vi "WPI_SerialPortGetPortName.vi"(8 "error in (no error)":errorcluster, 11 "Serial Port":T1) -> (0 "error out":errorcluster, 3 "VISA Refnum out":refnum<visa-resource-name>)   [LabVIEW 2017]
uses:
  <vilib>/Rock Robotics/WPI/SerialPort/WPI_SerialPort.ctl
panel:
  out "Hub Path":string[](array[string])
  out "OS Resource":string[](array[string])
  out "VISA Resource":string[](array[string])
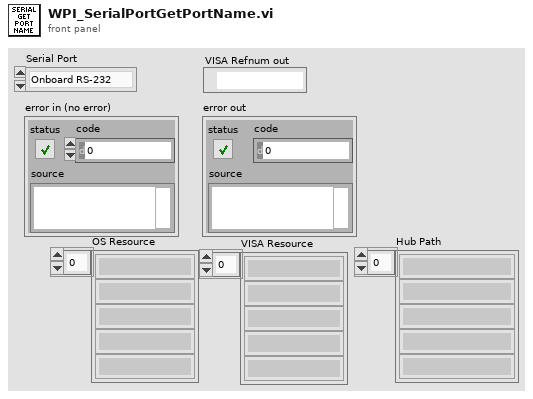
[diagram p1: front panel]
types:
  T1 = typedef "WPI_SerialPort.ctl" = enum16{"Onboard RS-232", "MXP TTL", "USB 1", "USB 2"}
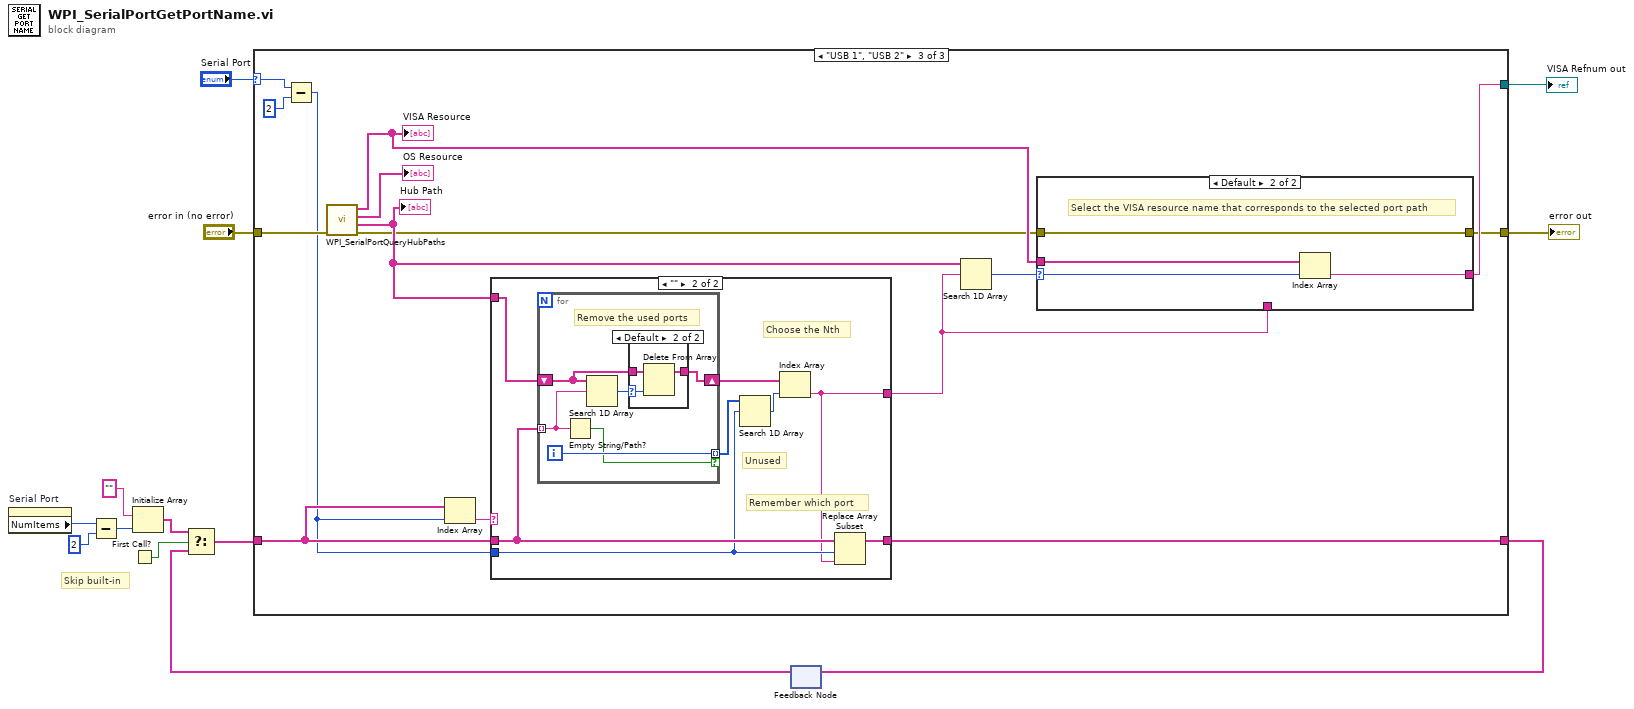
[diagram p0: block diagram]
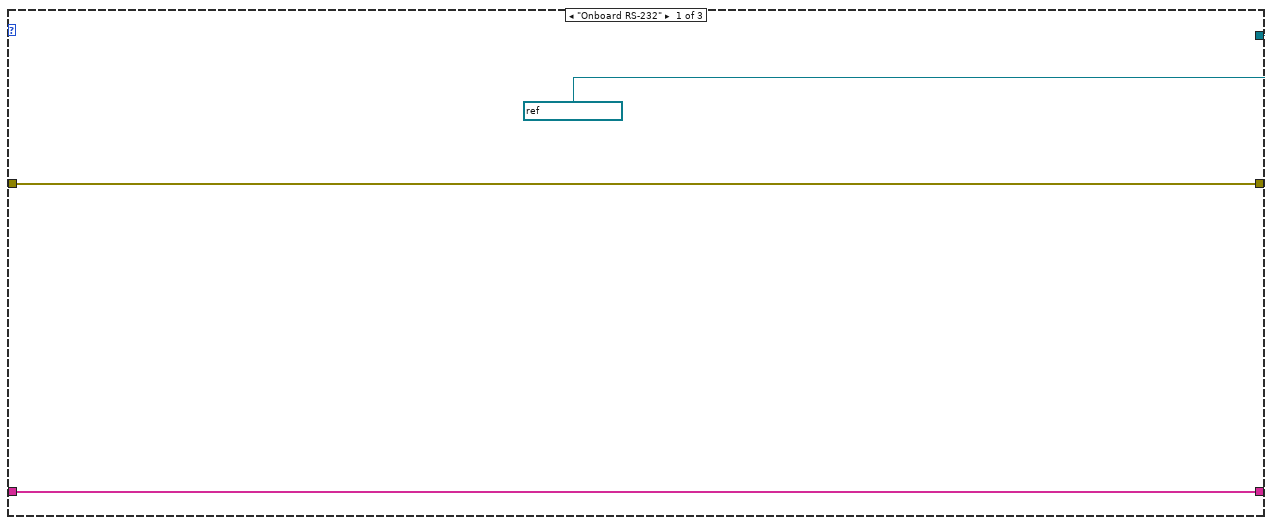
[diagram p2: hidden frame]
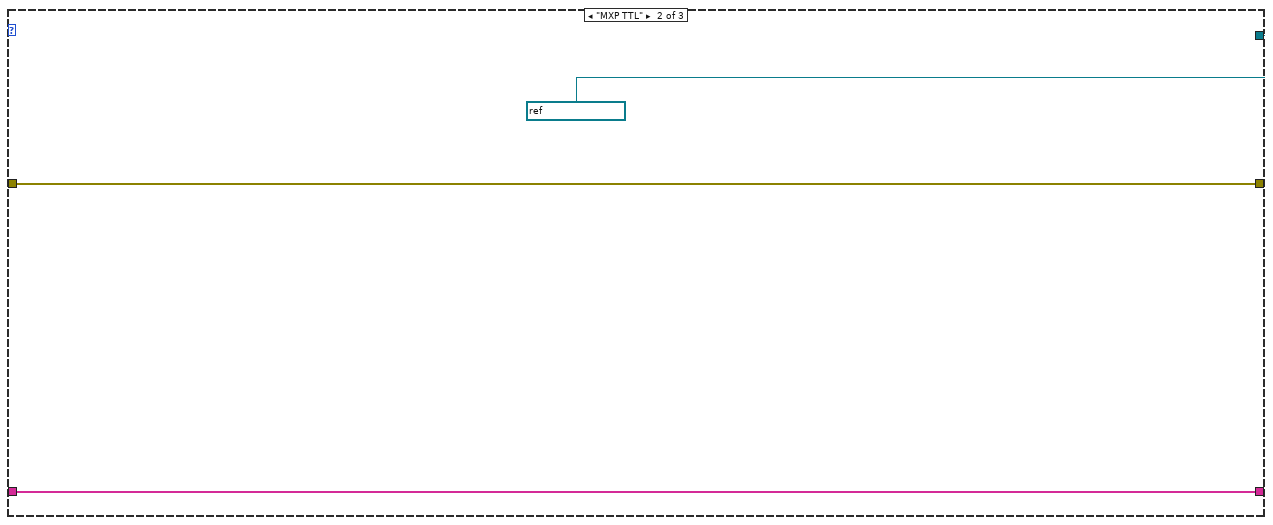
[diagram p3: hidden frame]
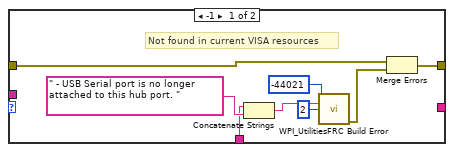
[diagram p4: hidden frame]
diagram:
  # "Skip built-in"
  n1 = property on="Serial Port" class="Enum (strict)"() -> ("NumItems"=w9:u32)  [unwired: 2 in, 2 out]
  n2 = Subtract(x=w9, y=u32 2 ("x")) -> (x-y=w2:u32)
  n3 = First Call?() -> (First Call?: T/F=w6:bool)
  n4 = Initialize Array("", w2) -> (w7:string[])
  n5 = feedback #1() -> (w5:string[])  [unwired: 1 in]
  n6 = Select(t=w7, s=w6, f=w5) -> (s? t:f=w4:string[])
  n7 = case shown="\"USB 1\", \"USB 2\"" "Serial Port" {
    selector: "Serial Port" -> [_ _ w29]
    tunnel: [refnum<visa-resource-name> "ASRL1::INSTR" ("VISA resource name") refnum<visa-resource-name> "ASRL2::INSTR" ("VISA resource name") w23] -> w13
    tunnel: "error in (no error)" -> [w15 w18 w34]
    tunnel: [w15 w18 w21] -> w10
    tunnel: w4 -> [w14 w17 w31]
    tunnel: [w14 w17 w27] -> w3
    frame "Onboard RS-232" {
    }
    frame "MXP TTL" {
    }
    frame "USB 1", "USB 2" {
      n8 = Subtract(x=w29, y=2 ("x")) -> (x-y=w28:i32)
      n9 = call <vilib>:"WPI_SerialPortQueryHubPaths.vi"("error in (no error)"=w34) -> ("error out"=w22:errorcluster, "Hub Path"=w26:string[], "OS Resource"=→"OS Resource":string[], "VISA Resource"=w24:string[])  [unwired: 7 in]
      "VISA Resource" <- w24
      "Hub Path" <- w26
      n10 = Index Array(array=w31, index=w28) -> (element=w32:string)
      n11 = case shown="\"\"" w32 {
        selector: w32 -> [w47 _]
        tunnel: w31 -> [w48 w53]
        tunnel: w26 -> [_ w50]
        tunnel: w28 -> [_ w52]
        tunnel: [w48 w51] -> w27
        tunnel: [w47 w49] -> w20
        frame Default {
          # "Previously assigned - just use it."
        }
        frame "" {
          # "Remember which port"
          # "Choose the Nth"
          # "Unused"
          n12 = for {
            tunnel: w53 -> [w60] mode=indexing
            tunnel: [w62] -> w56 mode=indexing if=w61
            shift-right: [w57] -> w55
            shift-left: w50 -> [w59]
            i -> [w62]
            # "Remove the used ports"
            n13 = Empty String/Path?(string/path=w60) -> (empty?=w61:bool)
            n14 = Search 1D Array(1D array=w59, element=w60) -> (index of element=w58:i32)  [unwired: 1 in]
            n15 = case shown="Default" w58 {
              selector: w58 -> [_ w65]
              tunnel: w59 -> [w63 w66]
              tunnel: [w63 w64] -> w57
              frame -1 {
              }
              frame Default {
                n16 = Delete From Array(array=w66, index=w65) -> (array with subset deleted=w64:string[])  [unwired: 1 in, 1 out]
              }
            }
          }
          n17 = Search 1D Array(1D array=w56, element=w52) -> (index of element=w54:i32)  [unwired: 1 in]
          n18 = Index Array(array=w55, index=w54) -> (element=w49:string)
          n19 = Replace Array Subset(array=w53, new element=w49, index=w52) -> (w51:string[])
        }
      }
      n20 = Search 1D Array(1D array=w26, element=w20) -> (index of element=w25:i32)  [unwired: 1 in]
      n21 = case shown="Default" w25 {
        selector: w25 -> [_ w46]
        tunnel: w24 -> [_ w45]
        tunnel: [_ w44] -> w23
        tunnel: [w41 w43] -> w21
        tunnel: w22 -> [w42 w43]
        tunnel: w20 -> [w36 _]
        frame -1 {
          # "Not found in current VISA resources"
          n22 = Concatenate Strings(w36, " - USB Serial port is no longer attached to this hub port. " ("extra error text")) -> (w37:string)
          n23 = call <vilib>:"WPI_UtilitiesFRC Build Error.vi"("error code"=-44021, "extra error text"=w37, "chain levels to remove (1)"=2) -> ("error out"=w35:errorcluster)  [unwired: 2 in, 10 out]
          n24 = Merge Errors(w42, w35) -> (w41:errorcluster)
        }
        frame Default {
          # "Select the VISA resource name that corresponds to the selected port path"
          n25 = Index Array(array=w45, index=w46) -> (element=w44:string)
        }
      }
    }
  }
  "VISA Refnum out" <- w13
  "error out" <- w10
  n26 = feedback-in #1(w3) -> ()
